vi "test TCX read (installed 71).vi"() -> ()   [LabVIEW 2011] (continued)
Degrees><LongitudeDegrees>-78.909779</LongitudeDegrees></Position><AltitudeMeters>75.120</AltitudeMeters><DistanceMeters>15266.510</DistanceMeters><Cadence>72</Cadence><Extensions><TPX xmlns=\"http://www.garmin.com/xmlschemas/ActivityExtension/v2\"><Watts>355</Watts></TPX></Extensions></Trackpoint><Trackpoint><Time>2008-03-03T23:13:11Z</Time><Position><LatitudeDegrees>35.863656</LatitudeDegrees><LongitudeDegrees>-78.909875</LongitudeDegrees></Position><AltitudeMeters>75.601</AltitudeMeters><DistanceMeters>15275.372</DistanceMeters><Cadence>73</Cadence><Extensions><TPX xmlns=\"http://www.garmin.com/xmlschemas/ActivityExtension/v2\"><Watts>375</Watts></TPX></Extensions></Trackpoint><Trackpoint><Time>2008-03-03T23:13:12Z</Time><Position><LatitudeDegrees>35.863672</LatitudeDegrees><LongitudeDegrees>-78.909971</LongitudeDegrees></Position><AltitudeMeters>75.120</AltitudeMeters><DistanceMeters>15284.272</DistanceMeters><Cadence>73</Cadence><Extensions><TPX xmlns=\"http://www.garmin.com/xmlschemas/ActivityExtension/v2\"><Watts>370</Watts></TPX></Extensions></Trackpoint><Trackpoint><Time>2008-03-03T23:13:13Z</Time><Position><LatitudeDegrees>35.863688</LatitudeDegrees><LongitudeDegrees>-78.910067</LongitudeDegrees></Position><AltitudeMeters>75.601</AltitudeMeters><DistanceMeters>15293.056</DistanceMeters><Cadence>72</Cadence><Extensions><TPX xmlns=\"http://www.garmin.com/xmlschemas/ActivityExtension/v2\"><Watts>375</Watts></TPX></Extensions></Trackpoint><Trackpoint><Time>2008-03-03T23:13:14Z</Time><Position><LatitudeDegrees>35.863704</LatitudeDegrees><LongitudeDegrees>-78.910161</LongitudeDegrees></Position><AltitudeMeters>76.562</AltitudeMeters><DistanceMeters>15301.760</DistanceMeters><Cadence>71</Cadence><Extensions><TPX xmlns=\"http://www.garmin.com/xmlschemas/ActivityExtension/v2\"><Watts>340</Watts></TPX></Extensions></Trackpoint><Trackpoint><Time>2008-03-03T23:13:15Z</Time><Position><LatitudeDegrees>35.863720</LatitudeDegrees><LongitudeDegrees>-78.910255</LongitudeDegrees></Position><AltitudeMeters>76.081</AltitudeMeters><DistanceMeters>15310.438</DistanceMeters><Cadence>70</Cadence><Extensions><TPX xmlns=\"http://www.garmin.com/xmlschemas/ActivityExtension/v2\"><Watts>338</Watts></TPX></Extensions></Trackpoint><Trackpoint><Time>2008-03-03T23:13:16Z</Time><Position><LatitudeDegrees>35.863737</LatitudeDegrees><LongitudeDegrees>-78.910348</LongitudeDegrees></Position><AltitudeMeters>76.562</AltitudeMeters><DistanceMeters>15319.036</DistanceMeters><Cadence>70</Cadence><Extensions><TPX xmlns=\"http://www.garmin.com/xmlschemas/ActivityExtension/v2\"><Watts>341</Watts></TPX></Extensions></Trackpoint><Trackpoint><Time>2008-03-03T23:13:17Z</Time><Position><LatitudeDegrees>35.863752</LatitudeDegrees><LongitudeDegrees>-78.910441</LongitudeDegrees></Position><AltitudeMeters>76.562</AltitudeMeters><DistanceMeters>15327.565</DistanceMeters><Cadence>70</Cadence><Extensions><TPX xmlns=\"http://www.garmin.com/xmlschemas/ActivityExtension/v2\"><Watts>349</Watts></TPX></Extensions></Trackpoint><Trackpoint><Time>2008-03-03T23:13:18Z</Time><Position><LatitudeDegrees>35.863768</LatitudeDegrees><LongitudeDegrees>-78.910533</LongitudeDegrees></Position><AltitudeMeters>77.043</AltitudeMeters><DistanceMeters>15336.047</DistanceMeters><Cadence>69</Cadence><Extensions><TPX xmlns=\"http://www.garmin.com/xmlschemas/ActivityExtension/v2\"><Watts>344</Watts></TPX></Extensions></Trackpoint><Trackpoint><Time>2008-03-03T23:13:19Z</Time><Position><LatitudeDegrees>35.863782</LatitudeDegrees><LongitudeDegrees>-78.910623</LongitudeDegrees></Position><AltitudeMeters>77.043</AltitudeMeters><DistanceMeters>15344.371</DistanceMeters><Cadence>69</Cadence><Extensions><TPX xmlns=\"http://www.garmin.com/xmlschemas/ActivityExtension/v2\"><Watts>327</Watts></TPX></Extensions></Trackpoint><Trackpoint><Time>2008-03-03T23:13:20Z</Time><Position><LatitudeDegrees>35.863796</LatitudeDegrees><LongitudeDegrees>-78.910714</LongitudeDegrees></Position><AltitudeMeters>77.043</AltitudeMeters><DistanceMeters>15352.690</DistanceMeters><Cadence>68</Cadence><Extensions><TPX xmlns=\"http://www.garmin.com/xmlschemas/ActivityExtension/v2\"><Watts>305</Watts></TPX></Extensions></Trackpoint><Trackpoint><Time>2008-03-03T23:13:21Z</Time><Position><LatitudeDegrees>35.863812</LatitudeDegrees><LongitudeDegrees>-78.910804</LongitudeDegrees></Position><AltitudeMeters>77.523</AltitudeMeters><DistanceMeters>15361.034</DistanceMeters><Cadence>68</Cadence><Extensions><TPX xmlns=\"http://www.garmin.com/xmlschemas/ActivityExtension/v2\"><Watts>301</Watts></TPX></Extensions></Trackpoint><Trackpoint><Time>2008-03-03T23:13:22Z</Time><Position><LatitudeDegrees>35.863828</LatitudeDegrees><LongitudeDegrees>-78.910893</LongitudeDegrees></Position><AltitudeMeters>77.523</AltitudeMeters><DistanceMeters>15369.291</DistanceMeters><Cadence>68</Cadence><Extensions><TPX xmlns=\"http://www.garmin.com/xmlschemas/ActivityExtension/v2\"><Watts>281</Watts></TPX></Extensions></Trackpoint><Trackpoint><Time>2008-03-03T23:13:23Z</Time><Position><LatitudeDegrees>35.863841</LatitudeDegrees><LongitudeDegrees>-78.910982</LongitudeDegrees></Position><AltitudeMeters>77.523</AltitudeMeters><DistanceMeters>15377.410</DistanceMeters><Cadence>67</Cadence><Extensions><TPX xmlns=\"http://www.garmin.com/xmlschemas/ActivityExtension/v2\"><Watts>292</Watts></TPX></Extensions></Trackpoint><Trackpoint><Time>2008-03-03T23:13:24Z</Time><Position><LatitudeDegrees>35.863856</LatitudeDegrees><LongitudeDegrees>-78.911071</LongitudeDegrees></Position><AltitudeMeters>78.004</AltitudeMeters><DistanceMeters>15385.608</DistanceMeters><Cadence>67</Cadence><Extensions><TPX xmlns=\"http://www.garmin.com/xmlschemas/ActivityExtension/v2\"><Watts>290</Watts></TPX></Extensions></Trackpoint><Trackpoint><Time>2008-03-03T23:13:25Z</Time><Position><LatitudeDegrees>35.863870</LatitudeDegrees><LongitudeDegrees>-78.911161</LongitudeDegrees></Position><AltitudeMeters>78.485</AltitudeMeters><DistanceMeters>15393.872</DistanceMeters><Cadence>68</Cadence><Extensions><TPX xmlns=\"http://www.garmin.com/xmlschemas/ActivityExtension/v2\"><Watts>287</Watts></TPX></Extensions></Trackpoint><Trackpoint><Time>2008-03-03T23:13:26Z</Time><Position><LatitudeDegrees>35.863885</LatitudeDegrees><LongitudeDegrees>-78.911251</LongitudeDegrees></Position><AltitudeMeters>78.485</AltitudeMeters><DistanceMeters>15402.214</DistanceMeters><Cadence>68</Cadence><Extensions><TPX xmlns=\"http://www.garmin.com/xmlschemas/ActivityExtension/v2\"><Watts>275</Watts></TPX></Extensions></Trackpoint><Trackpoint><Time>2008-03-03T23:13:27Z</Time><Position><LatitudeDegrees>35.863902</LatitudeDegrees><LongitudeDegrees>-78.911343</LongitudeDegrees></Position><AltitudeMeters>78.485</AltitudeMeters><DistanceMeters>15410.713</DistanceMeters><Cadence>69</Cadence><Extensions><TPX xmlns=\"http://www.garmin.com/xmlschemas/ActivityExtension/v2\"><Watts>275</Watts></TPX></Extensions></Trackpoint><Trackpoint><Time>2008-03-03T23:13:28Z</Time><Position><LatitudeDegrees>35.863918</LatitudeDegrees><LongitudeDegrees>-78.911434</LongitudeDegrees></Position><AltitudeMeters>78.485</AltitudeMeters><DistanceMeters>15419.151</DistanceMeters><Cadence>69</Cadence><Extensions><TPX xmlns=\"http://www.garmin.com/xmlschemas/ActivityExtension/v2\"><Watts>209</Watts></TPX></Extensions></Trackpoint><Trackpoint><Time>2008-03-03T23:13:29Z</Time><Position><LatitudeDegrees>35.863935</LatitudeDegrees><LongitudeDegrees>-78.911526</LongitudeDegrees></Position><AltitudeMeters>78.485</AltitudeMeters><DistanceMeters>15427.646</DistanceMeters><Cadence>69</Cadence><Extensions><TPX xmlns=\"http://www.garmin.com/xmlschemas/ActivityExtension/v2\"><Watts>211</Watts></TPX></Extensions></Trackpoint><Trackpoint><Time>2008-03-03T23:13:30Z</Time><Position><LatitudeDegrees>35.863952</LatitudeDegrees><LongitudeDegrees>-78.911617</LongitudeDegrees></Position><AltitudeMeters>78.965</AltitudeMeters><DistanceMeters>15436.117</DistanceMeters><Cadence>69</Cadence><Extensions><TPX xmlns=\"http://www.garmin.com/xmlschemas/ActivityExtension/v2\"><Watts>177</Watts></TPX></Extensions></Trackpoint><Trackpoint><Time>2008-03-03T23:13:31Z</Time><Position><LatitudeDegrees>35.863968</LatitudeDegrees><LongitudeDegrees>-78.911709</LongitudeDegrees></Position><AltitudeMeters>79.446</AltitudeMeters><DistanceMeters>15444.572</DistanceMeters><Cadence>69</Cadence><Extensions><TPX xmlns=\"http://www.garmin.com/xmlschemas/ActivityExtension/v2\"><Watts>160</Watts></TPX></Extensions></Trackpoint><Trackpoint><Time>2008-03-03T23:13:32Z</Time><Position><LatitudeDegrees>35.863984</LatitudeDegrees><LongitudeDegrees>-78.911801</LongitudeDegrees></Position><AltitudeMeters>78.965</AltitudeMeters><DistanceMeters>15453.188</DistanceMeters><Cadence>69</Cadence><Extensions><TPX xmlns=\"http://www.garmin.com/xmlschemas/ActivityExtension/v2\"><Watts>157</Watts></TPX></Extensions></Trackpoint><Trackpoint><Time>2008-03-03T23:13:33Z</Time><Position><LatitudeDegrees>35.864001</LatitudeDegrees><LongitudeDegrees>-78.911895</LongitudeDegrees></Position><AltitudeMeters>78.965</AltitudeMeters><DistanceMeters>15461.803</DistanceMeters><Cadence>71</Cadence><Extensions><TPX xmlns=\"http://www.garmin.com/xmlschemas/ActivityExtension/v2\"><Watts>155</Watts></TPX></Extensions></Trackpoint><Trackpoint><Time>2008-03-03T23:13:34Z</Time><Position><LatitudeDegrees>35.864018</LatitudeDegrees><LongitudeDegrees>-78.911990</LongitudeDegrees></Position><AltitudeMeters>78.965</AltitudeMeters><DistanceMeters>15470.562</DistanceMeters><Cadence>71</Cadence><Extensions><TPX xmlns=\"http://www.garmin.com/xmlschemas/ActivityExtension/v2\"><Watts>128</Watts></TPX></Extensions></Trackpoint><Trackpoint><Time>2008-03-03T23:13:35Z</Time><Position><LatitudeDegrees>35.864034</LatitudeDegrees><LongitudeDegrees>-78.912087</LongitudeDegrees></Position><AltitudeMeters>78.485</AltitudeMeters><DistanceMeters>15479.555</DistanceMeters><Cadence>74</Cadence><Extensions><TPX xmlns=\"http://www.garmin.com/xmlschemas/ActivityExtension/v2\"><Watts>83</Watts></TPX></Extensions></Trackpoint><Trackpoint><Time>2008-03-03T23:13:36Z</Time><Position><LatitudeDegrees>35.864051</LatitudeDegrees><LongitudeDegrees>-78.912188</LongitudeDegrees></Position><AltitudeMeters>78.004</AltitudeMeters><DistanceMeters>15488.854</DistanceMeters><Cadence>76</Cadence><Extensions><TPX xmlns=\"http://www.garmin.com/xmlschemas/ActivityExtension/v2\"><Watts>72</Watts></TPX></Extensions></Trackpoint><Trackpoint><Time>2008-03-03T23:13:37Z</Time><Position><LatitudeDegrees>35.864068</LatitudeDegrees><LongitudeDegrees>-78.912292</LongitudeDegrees></Position><AltitudeMeters>77.523</AltitudeMeters><DistanceMeters>15498.498</DistanceMeters><Cadence>78</Cadence><Extensions><TPX xmlns=\"http://www.garmin.com/xmlschemas/ActivityExtension/v2\"><Watts>68</Watts></TPX></Extensions></Trackpoint><Trackpoint><Time>2008-03-03T23:13:38Z</Time><Position><LatitudeDegrees>35.864086</LatitudeDegrees><LongitudeDegrees>-78.912401</LongitudeDegrees></Position><AltitudeMeters>76.562</AltitudeMeters><DistanceMeters>15508.492</DistanceMeters><Cadence>83</Cadence><Extensions><TPX xmlns=\"http://www.garmin.com/xmlschemas/ActivityExtension/v2\"><Watts>63</Watts></TPX></Extensions></Trackpoint><Trackpoint><Time>2008-03-03T23:13:39Z</Time><Position><LatitudeDegrees>35.864105</LatitudeDegrees><LongitudeDegrees>-78.912514</LongitudeDegrees></Position><AltitudeMeters>76.562</AltitudeMeters><DistanceMeters>15518.932</DistanceMeters><Cadence>83</Cadence><Extensions><TPX xmlns=\"http://www.garmin.com/xmlschemas/ActivityExtension/v2\"><Watts>59</Watts></TPX></Extensions></Trackpoint><Trackpoint><Time>2008-03-03T23:13:40Z</Time><Position><LatitudeDegrees>35.864125</LatitudeDegrees><LongitudeDegrees>-78.912631</LongitudeDegrees></Position><AltitudeMeters>76.081</AltitudeMeters><DistanceMeters>15529.836</DistanceMeters><Cadence>83</Cadence><Extensions><TPX xmlns=\"http://www.garmin.com/xmlschemas/ActivityExtension/v2\"><Watts>55</Watts></TPX></Extensions></Trackpoint><Trackpoint><Time>2008-03-03T23:13:41Z</Time><Position><LatitudeDegrees>35.864146</LatitudeDegrees><LongitudeDegrees>-78.912752</LongitudeDegrees></Position><AltitudeMeters>75.601</AltitudeMeters><DistanceMeters>15541.001</DistanceMeters><Cadence>80</Cadence><Extensions><TPX xmlns=\"http://www.garmin.com/xmlschemas/ActivityExtension/v2\"><Watts>55</Watts></TPX></Extensions></Trackpoint><Trackpoint><Time>2008-03-03T23:13:42Z</Time><Position><LatitudeDegrees>35.864167</LatitudeDegrees><LongitudeDegrees>-78.912877</LongitudeDegrees></Position><AltitudeMeters>75.120</AltitudeMeters><DistanceMeters>15552.565</DistanceMeters><Cadence>80</Cadence><Extensions><TPX xmlns=\"http://www.garmin.com/xmlschemas/ActivityExtension/v2\"><Watts>55</Watts></TPX></Extensions></Trackpoint><Trackpoint><Time>2008-03-03T23:13:43Z</Time><Position><LatitudeDegrees>35.864190</LatitudeDegrees><LongitudeDegrees>-78.913005</LongitudeDegrees></Position><AltitudeMeters>74.640</AltitudeMeters><DistanceMeters>15564.408</DistanceMeters><Cadence>86</Cadence><Extensions><TPX xmlns=\"http://www.garmin.com/xmlschemas/ActivityExtension/v2\"><Watts>70</Watts></TPX></Extensions></Trackpoint><Trackpoint><Time>2008-03-03T23:13:44Z</Time><Position><LatitudeDegrees>35.864213</LatitudeDegrees><LongitudeDegrees>-78.913141</LongitudeDegrees></Position><AltitudeMeters>73.678</AltitudeMeters><DistanceMeters>15577.016</DistanceMeters><Cadence>86</Cadence><Extensions><TPX xmlns=\"http://www.garmin.com/xmlschemas/ActivityExtension/v2\"><Watts>69</Watts></TPX></Extensions></Trackpoint><Trackpoint><Time>2008-03-03T23:13:45Z</Time><Position><LatitudeDegrees>35.864237</LatitudeDegrees><LongitudeDegrees>-78.913279</LongitudeDegrees></Position><AltitudeMeters>73.198</AltitudeMeters><DistanceMeters>15589.730</DistanceMeters><Cadence>91</Cadence><Extensions><TPX xmlns=\"http://www.garmin.com/xmlschemas/ActivityExtension/v2\"><Watts>83</Watts></TPX></Extensions></Trackpoint><Trackpoint><Time>2008-03-03T23:13:46Z</Time><Position><LatitudeDegrees>35.864259</LatitudeDegrees><LongitudeDegrees>-78.913419</LongitudeDegrees></Position><AltitudeMeters>72.236</AltitudeMeters><DistanceMeters>15602.657</DistanceMeters><Cadence>92</Cadence><Extensions><TPX xmlns=\"http://www.garmin.com/xmlschemas/ActivityExtension/v2\"><Watts>79</Watts></TPX></Extensions></Trackpoint><Trackpoint><Time>2008-03-03T23:13:47Z</Time><Position><LatitudeDegrees>35.864284</LatitudeDegrees><LongitudeDegrees>-78.913562</LongitudeDegrees></Position><AltitudeMeters>71.755</AltitudeMeters><DistanceMeters>15615.862</DistanceMeters><Cadence>93</Cadence><Extensions><TPX xmlns=\"http://www.garmin.com/xmlschemas/ActivityExtension/v2\"><Watts>79</Watts></TPX></Extensions></Trackpoint><Trackpoint><Time>2008-03-03T23:13:48Z</Time><Position><LatitudeDegrees>35.864308</LatitudeDegrees><LongitudeDegrees>-78.913706</LongitudeDegrees></Position><AltitudeMeters>71.755</AltitudeMeters><DistanceMeters>15629.100</DistanceMeters><Cadence>94</Cadence><Extensions><TPX xmlns=\"http://www.garmin.com/xmlschemas/ActivityExtension/v2\"><Watts>78</Watts></TPX></Extensions></Trackpoint><Trackpoint><Time>2008-03-03T23:13:49Z</Time><Position><LatitudeDegrees>35.864331</LatitudeDegrees><LongitudeDegrees>-78.913851</LongitudeDegrees></Position><AltitudeMeters>71.755</AltitudeMeters><DistanceMeters>15642.478</DistanceMeters><Cadence>94</Cadence><Extensions><TPX xmlns=\"http://www.garmin.com/xmlschemas/ActivityExtension/v2\"><Watts>77</Watts></TPX></Extensions></Trackpoint><Trackpoint><Time>2008-03-03T23:13:50Z</Time><Position><LatitudeDegrees>35.864353</LatitudeDegrees><LongitudeDegrees>-78.913997</LongitudeDegrees></Position><AltitudeMeters>71.755</AltitudeMeters><DistanceMeters>15655.923</DistanceMeters><Cadence>96</Cadence><Extensions><TPX xmlns=\"http://www.garmin.com/xmlschemas/ActivityExtension/v2\"><Watts>182</Watts></TPX></Extensions></Trackpoint><Trackpoint><Time>2008-03-03T23:13:51Z</Time><Position><LatitudeDegrees>35.864375</LatitudeDegrees><LongitudeDegrees>-78.914144</LongitudeDegrees></Position><AltitudeMeters>70.313</AltitudeMeters><DistanceMeters>15669.350</DistanceMeters><Cadence>97</Cadence><Extensions><TPX xmlns=\"http://www.garmin.com/xmlschemas/ActivityExtension/v2\"><Watts>210</Watts></TPX></Extensions></Trackpoint><Trackpoint><Time>2008-03-03T23:13:52Z</Time><Position><LatitudeDegrees>35.864398</LatitudeDegrees><LongitudeDegrees>-78.914291</LongitudeDegrees></Position><AltitudeMeters>69.833</AltitudeMeters><DistanceMeters>15683.004</DistanceMeters><Cadence>97</Cadence><Extensions><TPX xmlns=\"http://www.garmin.com/xmlschemas/ActivityExtension/v2\"><Watts>207</Watts></TPX></Extensions></Trackpoint><Trackpoint><Time>2008-03-03T23:13:53Z</Time><Position><LatitudeDegrees>35.864418</LatitudeDegrees><LongitudeDegrees>-78.914438</LongitudeDegrees></Position><AltitudeMeters>69.352</AltitudeMeters><DistanceMeters>15696.352</DistanceMeters><Cadence>96</Cadence><Extensions><TPX xmlns=\"http://www.garmin.com/xmlschemas/ActivityExtension/v2\"><Watts>120</Watts></TPX></Extensions></Trackpoint><Trackpoint><Time>2008-03-03T23:13:54Z</Time><Position><LatitudeDegrees>35.864438</LatitudeDegrees><LongitudeDegrees>-78.914584</LongitudeDegrees></Position><AltitudeMeters>68.391</AltitudeMeters><DistanceMeters>15709.704</DistanceMeters><Cadence>96</Cadence><Extensions><TPX xmlns=\"http://www.garmin.com/xmlschemas/ActivityExtension/v2\"><Watts>105</Watts></TPX></Extensions></Trackpoint><Trackpoint><Time>2008-03-03T23:13:55Z</Time><Position><LatitudeDegrees>35.864463</LatitudeDegrees><LongitudeDegrees>-78.914731</LongitudeDegrees></Position><AltitudeMeters>67.430</AltitudeMeters><DistanceMeters>15723.356</DistanceMeters><Cadence>95</Cadence><Extensions><TPX xmlns=\"http://www.garmin.com/xmlschemas/ActivityExtension/v2\"><Watts>102</Watts></TPX></Extensions></Trackpoint><Trackpoint><Time>2008-03-03T23:13:56Z</Time><Position><LatitudeDegrees>35.864489</LatitudeDegrees><LongitudeDegrees>-78.914876</LongitudeDegrees></Position><AltitudeMeters>67.430</AltitudeMeters><DistanceMeters>15736.706</DistanceMeters><Cadence>94</Cadence><Extensions><TPX xmlns=\"http://www.garmin.com/xmlschemas/ActivityExtension/v2\"><Watts>98</Watts></TPX></Extensions></Trackpoint><Trackpoint><Time>2008-03-03T23:13:57Z</Time><Position><LatitudeDegrees>35.864512</LatitudeDegrees><LongitudeDegrees>-78.915018</LongitudeDegrees></Position><AltitudeMeters>67.430</AltitudeMeters><DistanceMeters>15749.757</DistanceMeters><Cadence>91</Cadence><Extensions><TPX xmlns=\"http://www.garmin.com/xmlschemas/ActivityExtension/v2\"><Watts>87</Watts></TPX></Extensions></Trackpoint><Trackpoint><Time>2008-03-03T23:13:58Z</Time><Position><LatitudeDegrees>35.864541</LatitudeDegrees><LongitudeDegrees>-78.915155</LongitudeDegrees></Position><AltitudeMeters>66.949</AltitudeMeters><DistanceMeters>15762.511</DistanceMeters><Cadence>89</Cadence><Extensions><TPX xmlns=\"http://www.garmin.com/xmlschemas/ActivityExtension/v2\"><Watts>71</Watts></TPX></Extensions></Trackpoint><Trackpoint><Time>2008-03-03T23:13:59Z</Time><Position><LatitudeDegrees>35.864598</LatitudeDegrees><LongitudeDegrees>-78.915297</LongitudeDegrees></Position><AltitudeMeters>67.430</AltitudeMeters><DistanceMeters>15776.732</DistanceMeters><Cadence>89</Cadence><Extensions><TPX xmlns=\"http://www.garmin.com/xmlschemas/ActivityExtension/v2\"><Watts>72</Watts></TPX></Extensions></Trackpoint><Trackpoint><Time>2008-03-03T23:14:00Z</Time><Position><LatitudeDegrees>35.864677</LatitudeDegrees><LongitudeDegrees>-78.915398</LongitudeDegrees></Position><AltitudeMeters>66.949</AltitudeMeters><DistanceMeters>15789.389</DistanceMeters><Cadence>82</Cadence><Extensions><TPX xmlns=\"http://www.garmin.com/xmlschemas/ActivityExtension/v2\"><Watts>70</Watts></TPX></Extensions></Trackpoint><Trackpoint><Time>2008-03-03T23:14:01Z</Time><Position><LatitudeDegrees>35.864780</LatitudeDegrees><LongitudeDegrees>-78.915450</LongitudeDegrees></Position><AltitudeMeters>66.949</AltitudeMeters><DistanceMeters>15801.820</DistanceMeters><Cadence>82</Cadence><Extensions><TPX xmlns=\"http://www.garmin.com/xmlschemas/ActivityExtension/v2\"><Watts>71</Watts></TPX></Extensions></Trackpoint><Trackpoint><Time>2008-03-03T23:14:02Z</Time><Position><LatitudeDegrees>35.864884</LatitudeDegrees><LongitudeDegrees>-78.915465</LongitudeDegrees></Position><AltitudeMeters>66.949</AltitudeMeters><DistanceMeters>15813.393</DistanceMeters><Cadence>78</Cadence><Extensions><TPX xmlns=\"http://www.garmin.com/xmlschemas/ActivityExtension/v2\"><Watts>89</Watts></TPX></Extensions></Trackpoint><Trackpoint><Time>2008-03-03T23:14:03Z</Time><Position><LatitudeDegrees>35.864979</LatitudeDegrees><LongitudeDegrees>-78.915461</LongitudeDegrees></Position><AltitudeMeters>67.430</AltitudeMeters><DistanceMeters>15823.980</DistanceMeters><Cadence>72</Cadence><Extensions><TPX xmlns=\"http://www.garmin.com/xmlschemas/ActivityExtension/v2\"><Watts>155</Watts></TPX></Extensions></Trackpoint><Trackpoint><Time>2008-03-03T23:14:04Z</Time><Position><LatitudeDegrees>35.865070</LatitudeDegrees><LongitudeDegrees>-78.915448</LongitudeDegrees></Position><AltitudeMeters>67.430</AltitudeMeters><DistanceMeters>15834.147</DistanceMeters><Cadence>72</Cadence><Extensions><TPX xmlns=\"http://www.garmin.com/xmlschemas/ActivityExtension/v2\"><Watts>152</Watts></TPX></Extensions></Trackpoint><Trackpoint><Time>2008-03-03T23:14:05Z</Time><Position><LatitudeDegrees>35.865159</LatitudeDegrees><LongitudeDegrees>-78.915432</LongitudeDegrees></Position><AltitudeMeters>67.910</AltitudeMeters><DistanceMeters>15844.025</DistanceMeters><Cadence>80</Cadence><Extensions><TPX xmlns=\"http://www.garmin.com/xmlschemas/ActivityExtension/v2\"><Watts>176</Watts></TPX></Extensions></Trackpoint><Trackpoint><Time>2008-03-03T23:14:06Z</Time><Position><LatitudeDegrees>35.865246</LatitudeDegrees><LongitudeDegrees>-78.915418</LongitudeDegrees></Position><AltitudeMeters>68.391</AltitudeMeters><DistanceMeters>15853.817</DistanceMeters><Cadence>79</Cadence><Extensions><TPX xmlns=\"http://www.garmin.com/xmlschemas/ActivityExtension/v2\"><Watts>246</Watts></TPX></Extensions></Trackpoint><Trackpoint><Time>2008-03-03T23:14:07Z</Time><Position><LatitudeDegrees>35.865333</LatitudeDegrees><LongitudeDegrees>-78.915404</LongitudeDegrees></Position><AltitudeMeters>68.872</AltitudeMeters><DistanceMeters>15863.493</DistanceMeters><Cadence>79</Cadence><Extensions><TPX xmlns=\"http://www.garmin.com/xmlschemas/ActivityExtension/v2\"><Watts>371</Watts></TPX></Extensions></Trackpoint><Trackpoint><Time>2008-03-03T23:14:08Z</Time><Position><LatitudeDegrees>35.865418</LatitudeDegrees><LongitudeDegrees>-78.915391</LongitudeDegrees></Position><AltitudeMeters>68.872</AltitudeMeters><DistanceMeters>15873.026</DistanceMeters><Cadence>78</Cadence><Extensions><TPX xmlns=\"http://www.garmin.com/xmlschemas/ActivityExtension/v2\"><Watts>411</Watts></TPX></Extensions></Trackpoint><Trackpoint><Time>2008-03-03T23:14:09Z</Time><Position><LatitudeDegrees>35.865503</LatitudeDegrees><LongitudeDegrees>-78.915379</LongitudeDegrees></Position><AltitudeMeters>69.352</AltitudeMeters><DistanceMeters>15882.462</DistanceMeters><Cadence>78</Cadence><Extensions><TPX xmlns=\"http://www.garmin.com/xmlschemas/ActivityExtension/v2\"><Watts>418</Watts></TPX></Extensions></Trackpoint><Trackpoint><Time>2008-03-03T23:14:10Z</Time><Position><LatitudeDegrees>35.865587</LatitudeDegrees><LongitudeDegrees>-78.915368</LongitudeDegrees></Position><AltitudeMeters>69.833</AltitudeMeters><DistanceMeters>15891.883</DistanceMeters><Cadence>77</Cadence><Extensions><TPX xmlns=\"http://www.garmin.com/xmlschemas/ActivityExtension/v2\"><Watts>413</Watts></TPX></Extensions></Trackpoint><Trackpoint><Time>2008-03-03T23:14:11Z</Time><Position><LatitudeDegrees>35.865671</LatitudeDegrees><LongitudeDegrees>-78.915358</LongitudeDegrees></Position><AltitudeMeters>69.833</AltitudeMeters><DistanceMeters>15901.236</DistanceMeters><Cadence>77</Cadence><Extensions><TPX xmlns=\"http://www.garmin.com/xmlschemas/ActivityExtension/v2\"><Watts>415</Watts></TPX></Extensions></Trackpoint><Trackpoint><Time>2008-03-03T23:14:12Z</Time><Position><LatitudeDegrees>35.865755</LatitudeDegrees><LongitudeDegrees>-78.915347</LongitudeDegrees></Position><AltitudeMeters>69.833</AltitudeMeters><DistanceMeters>15910.614</DistanceMeters><Cadence>76</Cadence><Extensions><TPX xmlns=\"http://www.garmin.com/xmlschemas/ActivityExtension/v2\"><Watts>409</Watts></TPX></Extensions></Trackpoint><Trackpoint><Time>2008-03-03T23:14:13Z</Time><Position><LatitudeDegrees>35.865839</LatitudeDegrees><LongitudeDegrees>-78.915335</LongitudeDegrees></Position><AltitudeMeters>70.313</AltitudeMeters><DistanceMeters>15919.949</DistanceMeters><Cadence>76</Cadence><Extensions><TPX xmlns=\"http://www.garmin.com/xmlschemas/ActivityExtension/v2\"><Watts>394</Watts></TPX></Extensions></Trackpoint><Trackpoint><Time>2008-03-03T23:14:14Z</Time><Position><LatitudeDegrees>35.865917</LatitudeDegrees><LongitudeDegrees>-78.915329</LongitudeDegrees></Position><AltitudeMeters>70.313</AltitudeMeters><DistanceMeters>15928.672</DistanceMeters><Cadence>76</Cadence><Extensions><TPX xmlns=\"http://www.garmin.com/xmlschemas/ActivityExtension/v2\"><Watts>358</Watts></TPX></Extensions></Trackpoint><Trackpoint><Time>2008-03-03T23:14:15Z</Time><Position><LatitudeDegrees>35.865991</LatitudeDegrees><LongitudeDegrees>-78.915319</LongitudeDegrees></Position><AltitudeMeters>70.794</AltitudeMeters><DistanceMeters>15936.889</DistanceMeters><Cadence>76</Cadence><Extensions><TPX xmlns=\"http://www.garmin.com/xmlschemas/ActivityExtension/v2\"><Watts>334</Watts></TPX></Extensions></Trackpoint><Trackpoint><Time>2008-03-03T23:14:16Z</Time><Position><LatitudeDegrees>35.866070</LatitudeDegrees><LongitudeDegrees>-78.915303</LongitudeDegrees></Position><AltitudeMeters>70.794</AltitudeMeters><DistanceMeters>15945.708</DistanceMeters><Cadence>76</Cadence><Extensions><TPX xmlns=\"http://www.garmin.com/xmlschemas/ActivityExtension/v2\"><Watts>279</Watts></TPX></Extensions></Trackpoint><Trackpoint><Time>2008-03-03T23:14:17Z</Time><Position><LatitudeDegrees>35.866147</LatitudeDegrees><LongitudeDegrees>-78.915288</LongitudeDegrees></Position><AltitudeMeters>70.794</AltitudeMeters><DistanceMeters>15954.423</DistanceMeters><Cadence>77</Cadence><Extensions><TPX xmlns=\"http://www.garmin.com/xmlschemas/ActivityExtension/v2\"><Watts>165</Watts></TPX></Extensions></Trackpoint><Trackpoint><Time>2008-03-03T23:14:18Z</Time><Position><LatitudeDegrees>35.866233</LatitudeDegrees><LongitudeDegrees>-78.915263</LongitudeDegrees></Position><AltitudeMeters>70.794</AltitudeMeters><DistanceMeters>15964.225</DistanceMeters><Cadence>77</Cadence><Extensions><TPX xmlns=\"http://www.garmin.com/xmlschemas/ActivityExtension/v2\"><Watts>123</Watts></TPX></Extensions></Trackpoint><Trackpoint><Time>2008-03-03T23:14:19Z</Time><Position><LatitudeDegrees>35.866316</LatitudeDegrees><LongitudeDegrees>-78.915234</LongitudeDegrees></Position><AltitudeMeters>70.794</AltitudeMeters><DistanceMeters>15973.825</DistanceMeters><Cadence>78</Cadence><Extensions><TPX xmlns=\"http://www.garmin.com/xmlschemas/ActivityExtension/v2\"><Watts>102</Watts></TPX></Extensions></Trackpoint><Trackpoint><Time>2008-03-03T23:14:20Z</Time><Position><LatitudeDegrees>35.866402</LatitudeDegrees><LongitudeDegrees>-78.915200</LongitudeDegrees></Position><AltitudeMeters>70.794</AltitudeMeters><DistanceMeters>15983.826</DistanceMeters><Cadence>79</Cadence><Extensions><TPX xmlns=\"http://www.garmin.com/xmlschemas/ActivityExtension/v2\"><Watts>92</Watts></TPX></Extensions></Trackpoint><Trackpoint><Time>2008-03-03T23:14:21Z</Time><Position><LatitudeDegrees>35.866487</LatitudeDegrees><LongitudeDegrees>-78.915165</LongitudeDegrees></Position><AltitudeMeters>70.313</AltitudeMeters><DistanceMeters>15993.835</DistanceMeters><Cadence>81</Cadence><Extensions><TPX xmlns=\"http://www.garmin.com/xmlschemas/ActivityExtension/v2\"><Watts>93</Watts></TPX></Extensions></Trackpoint><Trackpoint><Time>2008-03-03T23:14:22Z</Time><Position><LatitudeDegrees>35.866574</LatitudeDegrees><LongitudeDegrees>-78.915122</LongitudeDegrees></Position><AltitudeMeters>69.833</AltitudeMeters><DistanceMeters>16004.274</DistanceMeters><Cadence>80</Cadence><Extensions><TPX xmlns=\"http://www.garmin.com/xmlschemas/ActivityExtension/v2\"><Watts>94</Watts></TPX></Extensions></Trackpoint><Trackpoint><Time>2008-03-03T23:14:23Z</Time><Position><LatitudeDegrees>35.866664</LatitudeDegrees><LongitudeDegrees>-78.915077</LongitudeDegrees></Position><AltitudeMeters>69.833</AltitudeMeters><DistanceMeters>16015.033</DistanceMeters><Cadence>80</Cadence><Extensions><TPX xmlns=\"http://www.garmin.com/xmlschemas/ActivityExtension/v2\"><Watts>102</Watts></TPX></Extensions></Trackpoint><Trackpoint><Time>2008-03-03T23:14:24Z</Time><Position><LatitudeDegrees>35.866755</LatitudeDegrees><LongitudeDegrees>-78.915031</LongitudeDegrees></Position><AltitudeMeters>69.833</AltitudeMeters><DistanceMeters>16025.952</DistanceMeters><Cadence>81</Cadence><Extensions><TPX xmlns=\"http://www.garmin.com/xmlschemas/ActivityExtension/v2\"><Watts>130</Watts></TPX></Extensions></Trackpoint><Trackpoint><Time>2008-03-03T23:14:25Z</Time><Position><LatitudeDegrees>35.866846</LatitudeDegrees><LongitudeDegrees>-78.914986</LongitudeDegrees></Position><AltitudeMeters>69.352</AltitudeMeters><DistanceMeters>16036.908</DistanceMeters><Cadence>83</Cadence><Extensions><TPX xmlns=\"http://www.garmin.com/xmlschemas/ActivityExtension/v2\"><Watts>153</Watts></TPX></Extensions></Trackpoint><Trackpoint><Time>2008-03-03T23:14:26Z</Time><Position><LatitudeDegrees>35.866941</LatitudeDegrees><LongitudeDegrees>-78.914941</LongitudeDegrees></Position><AltitudeMeters>68.872</AltitudeMeters><DistanceMeters>16048.229</DistanceMeters><Cadence>83</Cadence><Extensions><TPX xmlns=\"http://www.garmin.com/xmlschemas/ActivityExtension/v2\"><Watts>152</Watts></TPX></Extensions></Trackpoint><Trackpoint><Time>2008-03-03T23:14:27Z</Time><Position><LatitudeDegrees>35.867038</LatitudeDegrees><LongitudeDegrees>-78.914896</LongitudeDegrees></Position><AltitudeMeters>68.872</AltitudeMeters><DistanceMeters>16059.727</DistanceMeters><Cadence>88</Cadence><Extensions><TPX xmlns=\"http://www.garmin.com/xmlschemas/ActivityExtension/v2\"><Watts>200</Watts></TPX></Extensions></Trackpoint><Trackpoint><Time>2008-03-03T23:14:28Z</Time><Position><LatitudeDegrees>35.867136</LatitudeDegrees><LongitudeDegrees>-78.914850</LongitudeDegrees></Position><AltitudeMeters>68.872</AltitudeMeters><DistanceMeters>16071.396</DistanceMeters><Cadence>89</Cadence><Extensions><TPX xmlns=\"http://www.garmin.com/xmlschemas/ActivityExtension/v2\"><Watts>159</Watts></TPX></Extensions></Trackpoint><Trackpoint><Time>2008-03-03T23:14:29Z</Time><Position><LatitudeDegrees>35.867236</LatitudeDegrees><LongitudeDegrees>-78.914808</LongitudeDegrees></Position><AltitudeMeters>68.872</AltitudeMeters><DistanceMeters>16083.110</DistanceMeters><Cadence>89</Cadence><Extensions><TPX xmlns=\"http://www.garmin.com/xmlschemas/ActivityExtension/v2\"><Watts>158</Watts></TPX></Extensions></Trackpoint><Trackpoint><Time>2008-03-03T23:14:30Z</Time><Position><LatitudeDegrees>35.867336</LatitudeDegrees><LongitudeDegrees>-78.914774</LongitudeDegrees></Position><AltitudeMeters>68.391</AltitudeMeters><DistanceMeters>16094.578</DistanceMeters><Cadence>89</Cadence><Extensions><TPX xmlns=\"http://www.garmin.com/xmlschemas/ActivityExtension/v2\"><Watts>142</Watts></TPX></Extensions></Trackpoint><Trackpoint><Time>2008-03-03T23:14:31Z</Time><Position><LatitudeDegrees>35.867437</LatitudeDegrees><LongitudeDegrees>-78.914748</LongitudeDegrees></Position><AltitudeMeters>69.352</AltitudeMeters><DistanceMeters>16106.026</DistanceMeters><Cadence>89</Cadence><Extensions><TPX xmlns=\"http://www.garmin.com/xmlschemas/ActivityExtension/v2\"><Watts>140</Watts></TPX></Extensions></Trackpoint><Trackpoint><Time>2008-03-03T23:14:32Z</Time><Position><LatitudeDegrees>35.867539</LatitudeDegrees><LongitudeDegrees>-78.914733</LongitudeDegrees></Position><AltitudeMeters>69.352</AltitudeMeters><DistanceMeters>16117.415</DistanceMeters><Cadence>88</Cadence><Extensions><TPX xmlns=\"http://www.garmin.com/xmlschemas/ActivityExtension/v2\"><Watts>109</Watts></TPX></Extensions></Trackpoint><Trackpoint><Time>2008-03-03T23:14:33Z</Time><Position><LatitudeDegrees>35.867642</LatitudeDegrees><LongitudeDegrees>-78.914725</LongitudeDegrees></Position><AltitudeMeters>68.391</AltitudeMeters><DistanceMeters>16128.910</DistanceMeters><Cadence>88</Cadence><Extensions><TPX xmlns=\"http://www.garmin.com/xmlschemas/ActivityExtension/v2\"><Watts>102</Watts></TPX></Extensions></Trackpoint><Trackpoint><Time>2008-03-03T23:14:34Z</Time><Position><LatitudeDegrees>35.867744</LatitudeDegrees><LongitudeDegrees>-78.914721</LongitudeDegrees></Position><AltitudeMeters>69.352</AltitudeMeters><DistanceMeters>16140.199</DistanceMeters><Cadence>87</Cadence><Extensions><TPX xmlns=\"http://www.garmin.com/xmlschemas/ActivityExtension/v2\"><Watts>106</Watts></TPX></Extensions></Trackpoint><Trackpoint><Time>2008-03-03T23:14:35Z</Time><Position><LatitudeDegrees>35.867848</LatitudeDegrees><LongitudeDegrees>-78.914721</LongitudeDegrees></Position><AltitudeMeters>68.872</AltitudeMeters><DistanceMeters>16151.673</DistanceMeters><Cadence>87</Cadence><Extensions><TPX xmlns=\"http://www.garmin.com/xmlschemas/ActivityExtension/v2\"><Watts>111</Watts></TPX></Extensions></Trackpoint><Trackpoint><Time>2008-03-03T23:14:36Z</Time><Position><LatitudeDegrees>35.867952</LatitudeDegrees><LongitudeDegrees>-78.914720</LongitudeDegrees></Position><AltitudeMeters>68.391</AltitudeMeters><DistanceMeters>16163.203</DistanceMeters><Cadence>87</Cadence><Extensions><TPX xmlns=\"http://www.garmin.com/xmlschemas/ActivityExtension/v2\"><Watts>116</Watts></TPX></Extensions></Trackpoint><Trackpoint><Time>2008-03-03T23:14:37Z</Time><Position><LatitudeDegrees>35.868053</LatitudeDegrees><LongitudeDegrees>-78.914720</LongitudeDegrees></Position><AltitudeMeters>68.391</AltitudeMeters><DistanceMeters>16174.526</DistanceMeters><Cadence>87</Cadence><Extensions><TPX xmlns=\"http://www.garmin.com/xmlschemas/ActivityExtension/v2\"><Watts>127</Watts></TPX></Extensions></Trackpoint><Trackpoint><Time>2008-03-03T23:14:38Z</Time><Position><LatitudeDegrees>35.868156</LatitudeDegrees><LongitudeDegrees>-78.914718</LongitudeDegrees></Position><AltitudeMeters>68.391</AltitudeMeters><DistanceMeters>16185.894</DistanceMeters><Cadence>87</Cadence><Extensions><TPX xmlns=\"http://www.garmin.com/xmlschemas/ActivityExtension/v2\"><Watts>126</Watts></TPX></Extensions></Trackpoint><Trackpoint><Time>2008-03-03T23:14:39Z</Time><Position><LatitudeDegrees>35.868259</LatitudeDegrees><LongitudeDegrees>-78.914715</LongitudeDegrees></Position><AltitudeMeters>68.391</AltitudeMeters><DistanceMeters>16197.301</DistanceMeters><Cadence>85</Cadence><Extensions><TPX xmlns=\"http://www.garmin.com/xmlschemas/ActivityExtension/v2\"><Watts>145</Watts></TPX></Extensions></Trackpoint><Trackpoint><Time>2008-03-03T23:14:40Z</Time><Position><LatitudeDegrees>35.868361</LatitudeDegrees><LongitudeDegrees>-78.914712</LongitudeDegrees></Position><AltitudeMeters>67.910</AltitudeMeters><DistanceMeters>16208.585</DistanceMeters><Cadence>85</Cadence><Extensions><TPX xmlns=\"http://www.garmin.com/xmlschemas/ActivityExtension/v2\"><Watts>163</Watts></TPX></Extensions></Trackpoint><Trackpoint><Time>2008-03-03T23:14:41Z</Time><Position><LatitudeDegrees>35.868462</LatitudeDegrees><LongitudeDegrees>-78.914709</LongitudeDegrees></Position><AltitudeMeters>67.910</AltitudeMeters><DistanceMeters>16219.852</DistanceMeters><Cadence>85</Cadence><Extensions><TPX xmlns=\"http://www.garmin.com/xmlschemas/ActivityExtension/v2\"><Watts>166</Watts></TPX></Extensions></Trackpoint><Trackpoint><Time>2008-03-03T23:14:42Z</Time><Position><LatitudeDegrees>35.868563</LatitudeDegrees><LongitudeDegrees>-78.914707</LongitudeDegrees></Position><AltitudeMeters>67.910</AltitudeMeters><DistanceMeters>16231.049</DistanceMeters><Cadence>84</Cadence><Extensions><TPX xmlns=\"http://www.garmin.com/xmlschemas/ActivityExtension/v2\"><Watts>152</Watts></TPX></Extensions></Trackpoint><Trackpoint><Time>2008-03-03T23:14:43Z</Time><Position><LatitudeDegrees>35.868663</LatitudeDegrees><LongitudeDegrees>-78.914703</LongitudeDegrees></Position><AltitudeMeters>67.910</AltitudeMeters><DistanceMeters>16242.091</DistanceMeters><Cadence>83</Cadence><Extensions><TPX xmlns=\"http://www.garmin.com/xmlschemas/ActivityExtension/v2\"><Watts>135</Watts></TPX></Extensions></Trackpoint><Trackpoint><Time>2008-03-03T23:14:44Z</Time><Position><LatitudeDegrees>35.868762</LatitudeDegrees><LongitudeDegrees>-78.914697</LongitudeDegrees></Position><AltitudeMeters>67.910</AltitudeMeters><DistanceMeters>16253.078</DistanceMeters><Cadence>83</Cadence><Extensions><TPX xmlns=\"http://www.garmin.com/xmlschemas/ActivityExtension/v2\"><Watts>137</Watts></TPX></Extensions></Trackpoint><Trackpoint><Time>2008-03-03T23:14:45Z</Time><Position><LatitudeDegrees>35.868860</LatitudeDegrees><LongitudeDegrees>-78.914689</LongitudeDegrees></Position><AltitudeMeters>67.430</AltitudeMeters><DistanceMeters>16264.040</DistanceMeters><Cadence>83</Cadence><Extensions><TPX xmlns=\"http://www.garmin.com/xmlschemas/ActivityExtension/v2\"><Watts>141</Watts></TPX></Extensions></Trackpoint><Trackpoint><Time>2008-03-03T23:14:46Z</Time><Position><LatitudeDegrees>35.868958</LatitudeDegrees><LongitudeDegrees>-78.914677</LongitudeDegrees></Position><AltitudeMeters>67.430</AltitudeMeters><DistanceMeters>16274.903</DistanceMeters><Cadence>82</Cadence><Extensions><TPX xmlns=\"http://www.garmin.com/xmlschemas/ActivityExtension/v2\"><Watts>155</Watts></TPX></Extensions></Trackpoint><Trackpoint><Time>2008-03-03T23:14:47Z</Time><Position><LatitudeDegrees>35.869053</LatitudeDegrees><LongitudeDegrees>-78.914662</LongitudeDegrees></Position><AltitudeMeters>67.430</AltitudeMeters><DistanceMeters>16285.515</DistanceMeters><Cadence>82</Cadence><Extensions><TPX xmlns=\"http://www.garmin.com/xmlschemas/ActivityExtension/v2\"><Watts>155</Watts></TPX></Extensions></Trackpoint><Trackpoint><Time>2008-03-03T23:14:48Z</Time><Position><LatitudeDegrees>35.869148</LatitudeDegrees><LongitudeDegrees>-78.914643</LongitudeDegrees></Position><AltitudeMeters>67.430</AltitudeMeters><DistanceMeters>16296.295</DistanceMeters><Cadence>82</Cadence><Extensions><TPX xmlns=\"http://www.garmin.com/xmlschemas/ActivityExtension/v2\"><Watts>154</Watts></TPX></Extensions></Trackpoint><Trackpoint><Time>2008-03-03T23:14:49Z</Time><Position><LatitudeDegrees>35.869243</LatitudeDegrees><LongitudeDegrees>-78.914620</LongitudeDegrees></Position><AltitudeMeters>67.910</AltitudeMeters><DistanceMeters>16306.994</DistanceMeters><Cadence>80</Cadence><Extensions><TPX xmlns=\"http://www.garmin.com/xmlschemas/ActivityExtension/v2\"><Watts>181</Watts></TPX></Extensions></Trackpoint><Trackpoint><Time>2008-03-03T23:14:50Z</Time><Position><LatitudeDegrees>35.869337</LatitudeDegrees><LongitudeDegrees>-78.914590</LongitudeDegrees></Position><AltitudeMeters>67.430</AltitudeMeters><DistanceMeters>16317.800</DistanceMeters><Cadence>80</Cadence><Extensions><TPX xmlns=\"http://www.garmin.com/xmlschemas/ActivityExtension/v2\"><Watts>181</Watts></TPX></Extensions></Trackpoint><Trackpoint><Time>2008-03-03T23:14:51Z</Time><Position><LatitudeDegrees>35.869429</LatitudeDegrees><LongitudeDegrees>-78.914555</LongitudeDegrees></Position><AltitudeMeters>67.430</AltitudeMeters><DistanceMeters>16328.455</DistanceMeters><Cadence>80</Cadence><Extensions><TPX xmlns=\"http://www.garmin.com/xmlschemas/ActivityExtension/v2\"><Watts>162</Watts></TPX></Extensions></Trackpoint><Trackpoint><Time>2008-03-03T23:14:52Z</Time><Position><LatitudeDegrees>35.869519</LatitudeDegrees><LongitudeDegrees>-78.914516</LongitudeDegrees></Position><AltitudeMeters>67.910</AltitudeMeters><DistanceMeters>16339.045</DistanceMeters><Cadence>80</Cadence><Extensions><TPX xmlns=\"http://www.garmin.com/xmlschemas/ActivityExtension/v
